vi "Apply Angular Velocity.vi"(8 "error in (no error)":errorcluster, 10 "forward angular velocity":dbl, 11 "wheel in":refnum<class "NI_Robotics_Wheel.lvclass">) -> (0 "error out":errorcluster, 3 "wheel out":refnum<class "NI_Robotics_Wheel.lvclass">)   [LabVIEW 2017, in "NI_Robotics_Wheel.lvclass"]
uses:
  <vilib>/robotics/Steering/Wheel/NI_Robotics_Wheel.lvclass
  <vilib>/robotics/Steering/Wheel/NI_Robotics_Wheel.lvclass/NI_Robotics_Wheel.ctl
  <vilib>/robotics/Actuation/Motor Communication/Check if Valid.vi
  <vilib>/robotics/Utilities/Generate Error.vi
  <vilib>/robotics/Actuation/Motor Communication/NI_Robotics_Motor Communication.lvclass
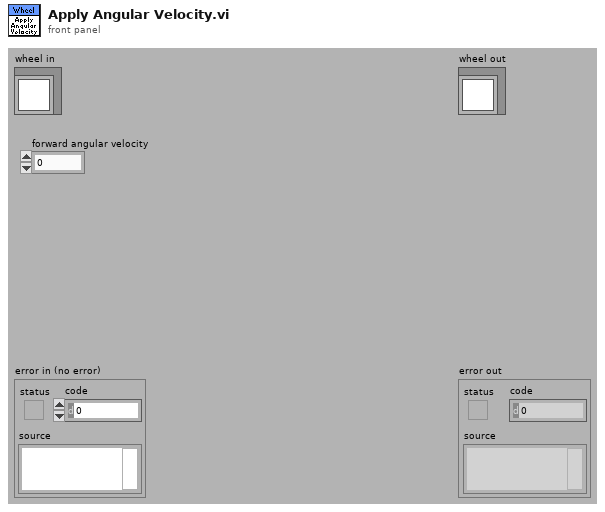
[diagram p1: front panel]
types:
  T1 = typedef "NI_Robotics_Wheel.lvclass/Rotation Direction.ctl" = u16
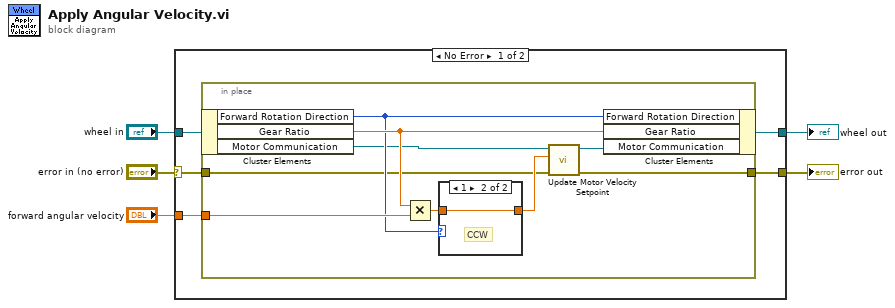
[diagram p0: block diagram]
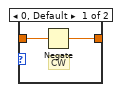
[diagram p2: hidden frame]
diagram:
  n1 = case shown="No Error" "error in (no error)" {
    selector: "error in (no error)" -> [w9 w24]
    tunnel: [w6 w24] -> w4
    tunnel: [w8 w23] -> w2
    tunnel: "wheel in" -> [w10 w23]
    tunnel: "forward angular velocity" -> [w7 _]
    frame No Error {
      n2 = in-place {
        in-place-border: w9 -> [w12]
        in-place-border: w7 -> [w18]
        in-place-border: [w11] -> w6
        n3 = in-place-cluster #1(w10) -> ("Forward Rotation Direction"=w16:T1, "Gear Ratio"=w19:dbl, "Motor Communication"=w14:refnum<class "NI_Robotics_Motor Communication.lvclass">)
        n4 = Multiply(x=w19, y=w18) -> (x*y=w17:dbl)
        n5 = case shown="1" w16 {
          tunnel: w17 -> [w21 w22]
          tunnel: [w20 w22] -> w15
          frame 0, Default {
            # "CW"
            n6 = Negate(x=w21) -> (-x=w20:dbl)
          }
          frame 1 {
            # "CCW"
          }
        }
        n7 = call <vilib>:"Update Motor Velocity Setpoint.vi"("error in (no error)"=w12, "velocity"=w15, "motor communication in"=w14) -> ("error out"=w11:errorcluster, "motor communication out"=w13:refnum<class "NI_Robotics_Motor Communication.lvclass">)  [unwired: 6 in, 1 out]
        n8 = in-place-cluster #1("Forward Rotation Direction"=w16, "Gear Ratio"=w19, "Motor Communication"=w13) -> (w8:refnum<class "NI_Robotics_Wheel.lvclass">)
      }
    }
    frame Error {
    }
  }
  "error out" <- w4
  "wheel out" <- w2
